vi "Logout_init.vi"(8 "error in (no error)":errorcluster, 11 "ZenGage v3.0 UI in":T1) -> (0 "error out":errorcluster)   [LabVIEW 2019, in "ZenGage v3.0 UI.lvclass"]
uses:
  ZenGage v3.0 UI.lvclass
  <vilib>/Utility/miscctls.llb/LVRowAndColumnTypeDef.ctl
  Type Definitions/Controls and Indicators/Select a part (combobox).ctl
  Type Definitions/Controls and Indicators/EDL control references.ctl
  Type Definitions/Controls and Indicators/Diagnostics control referencs.ctl
  Type Definitions/Controls and Indicators/Inspection control references.ctl
  Type Definitions/Controls and Indicators/General_Control references.ctl
  Type Definitions/Controls and Indicators/Controls and Indicators Cluster.ctl
  Type Definitions/General/Master sample references.ctl
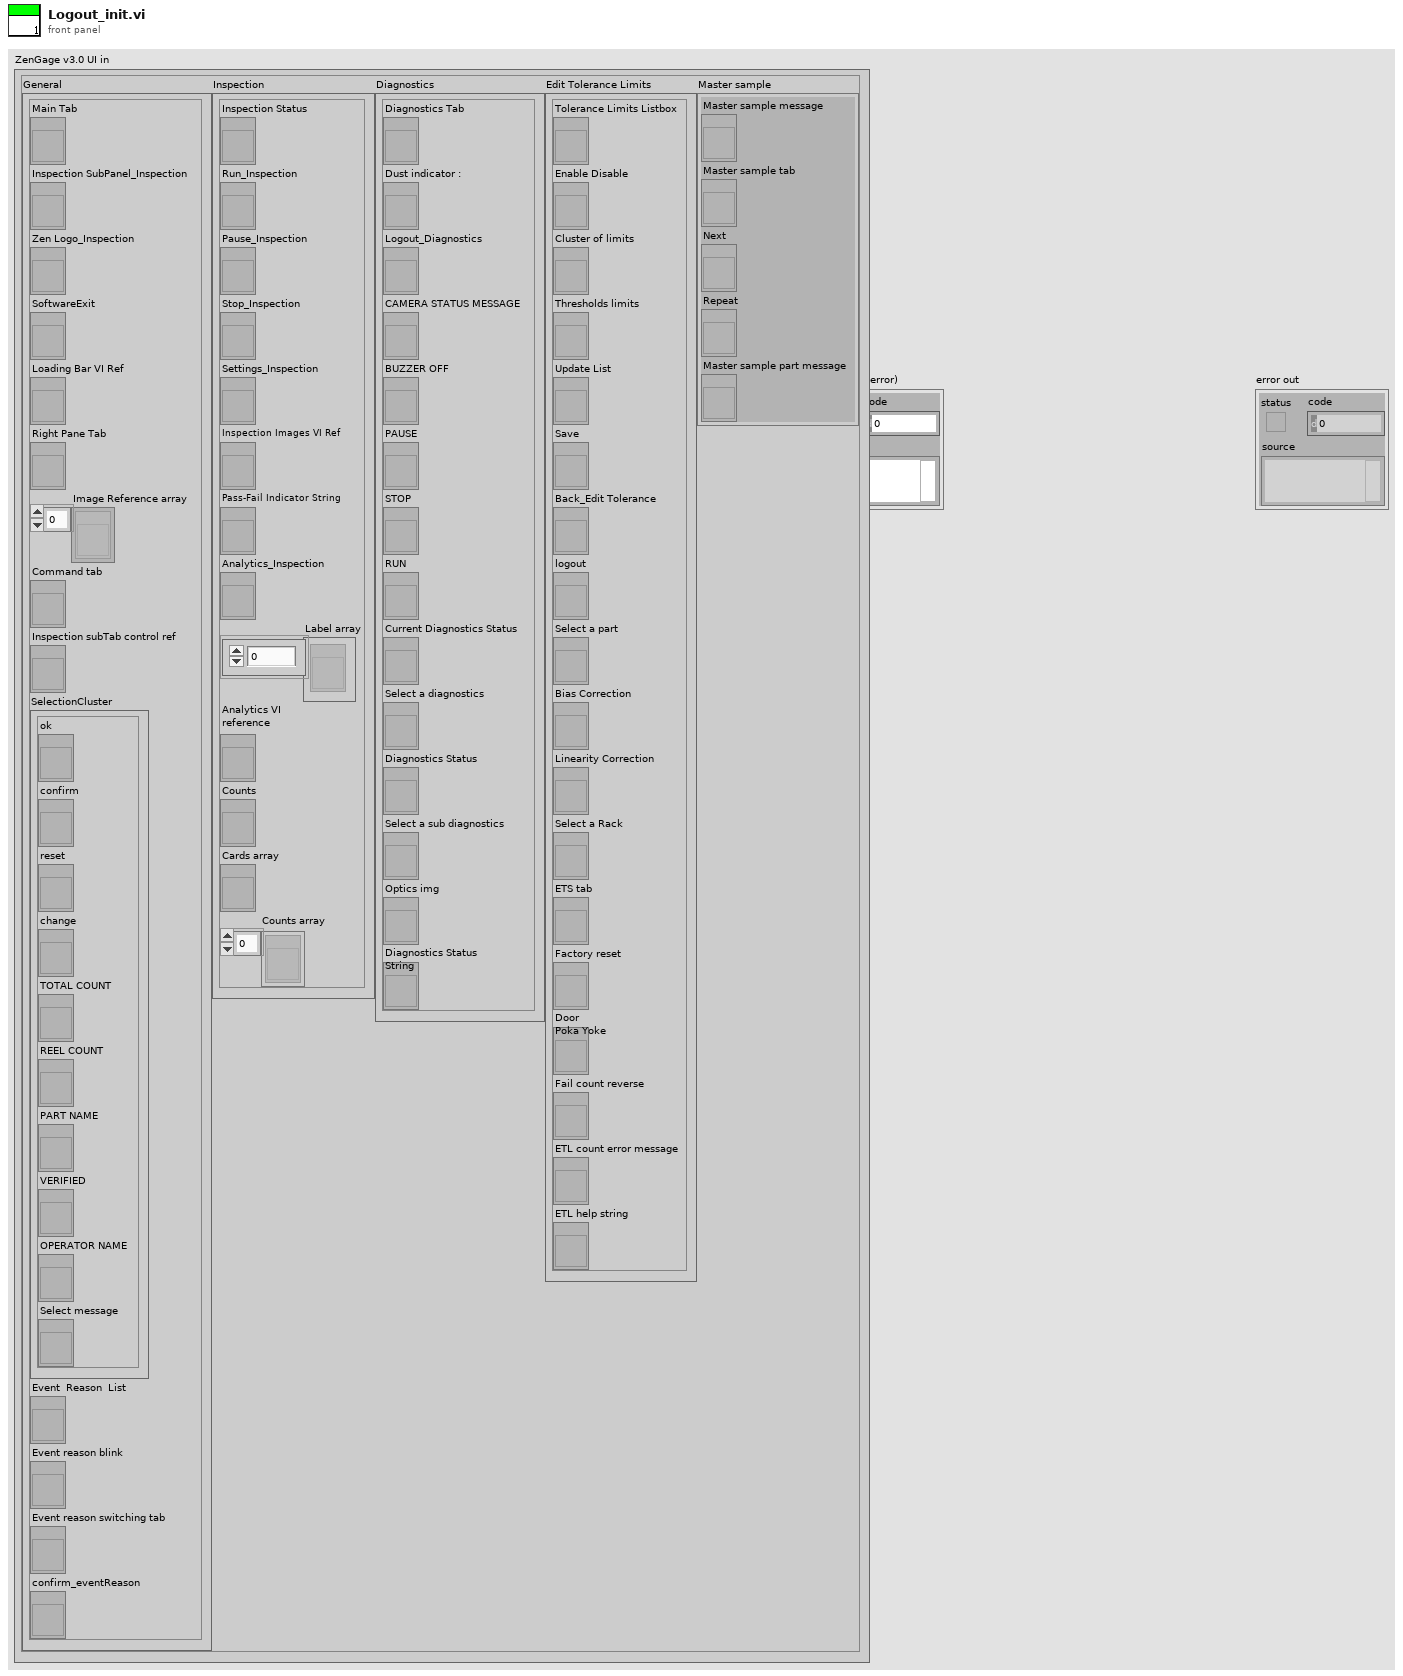
[diagram p1: front panel]
types:
  T1 = typedef "ZenGage v3.0 UI.lvclass/Controls and Indicators Cluster.ctl" = cluster{"General":T2, "Inspection":T3, "Diagnostics":T4, "Edit Tolerance Limits":T5, "Master sample":T6}
  T2 = typedef "ZenGage v3.0 UI.lvclass/General_Control references.ctl" = cluster{"Main Tab":refnum<vi>, "Inspection SubPanel_Inspection":refnum<vi>, "Zen Logo_Inspection":refnum<vi>, "SoftwareExit":refnum<vi>, "Loading Bar VI Ref":refnum<vi>, "Right Pane Tab":refnum<vi>, "Image Reference array":refnum<vi>[], "Command tab":refnum<vi>, "Inspection subTab control ref":refnum<vi>, "SelectionCluster":cluster{"ok":refnum<vi>, "confirm":refnum<vi>, "reset":refnum<vi>, "change":refnum<vi>, "TOTAL COUNT":refnum<vi>, "REEL COUNT":refnum<vi>, "PART NAME":refnum<vi>, "VERIFIED":refnum<vi>, "OPERATOR NAME":refnum<vi>, "Select message":refnum<vi>}, "Event  Reason  List":refnum<vi>, "Event reason blink":refnum<vi>, "Event reason switching tab":refnum<vi>, "confirm_eventReason":refnum<vi>}
  T3 = typedef "ZenGage v3.0 UI.lvclass/Inspection control references.ctl" = cluster{"Inspection Status":refnum<vi>, "Run_Inspection":refnum<vi>, "Pause_Inspection":refnum<vi>, "Stop_Inspection":refnum<vi>, "Settings_Inspection":refnum<vi>, "Inspection Images VI Ref":refnum<vi>, "Pass-Fail Indicator String":refnum<vi>, "Analytics_Inspection":refnum<vi>, "Label array":refnum<vi>[], "Analytics VI\nreference":refnum<vi>, "Counts":refnum<vi>, "Cards array":refnum<vi>, "Counts array":refnum<vi>[]}
  T4 = typedef "ZenGage v3.0 UI.lvclass/Diagnostics control referencs.ctl" = cluster{"Diagnostics Tab":refnum<vi>, "Dust indicator :":refnum<vi>, "Logout_Diagnostics":refnum<vi>, "CAMERA STATUS MESSAGE":refnum<vi>, "BUZZER OFF":refnum<vi>, "PAUSE":refnum<vi>, "STOP":refnum<vi>, "RUN":refnum<vi>, "Current Diagnostics Status":refnum<vi>, "Select a diagnostics":refnum<vi>, "Diagnostics Status":refnum<vi>, "Select a sub diagnostics":refnum<vi>, "Optics img":refnum<vi>, "Diagnostics Status\nString":refnum<vi>}
  T5 = typedef "ZenGage v3.0 UI.lvclass/EDL control references.ctl" = cluster{"Tolerance Limits Listbox":refnum<vi>, "Enable Disable":refnum<vi>, "Cluster of limits":refnum<vi>, "Thresholds limits":refnum<vi>, "Update List":refnum<vi>, "Save":refnum<vi>, "Back_Edit Tolerance":refnum<vi>, "logout":refnum<vi>, "Select a part":refnum<vi>, "Bias Correction":refnum<vi>, "Linearity Correction":refnum<vi>, "Select a Rack":refnum<vi>, "ETS tab":refnum<vi>, "Factory reset":refnum<vi>, "Door\nPoka Yoke":refnum<vi>, "Fail count reverse":refnum<vi>, "ETL count error message":refnum<vi>, "ETL help string":refnum<vi>}
  T6 = typedef "Master sample references.ctl" = cluster{"Master sample message":refnum<vi>, "Master sample tab":refnum<vi>, "Next":refnum<vi>, "Repeat":refnum<vi>, "Master sample part message":refnum<vi>}
  T7 = enum32{"Edit Tolerance Limits1", "Inspection", "Master sample", "Diagnostics"}
  T8 = enum32{"Arduino Motor", "Sensor trigger", "Hardware Button", "Camera Optics"}
  T9 = enum8{"Enabled", "Disabled", "Disabled and Grayed Out"}
  T10 = enum32{"Inspection", "Diagnostics", "Edit Tolerance Settings"}
  T11 = typedef "LVRowAndColumnTypeDef.ctl" = cluster{"Row":i32, "Column":i32}
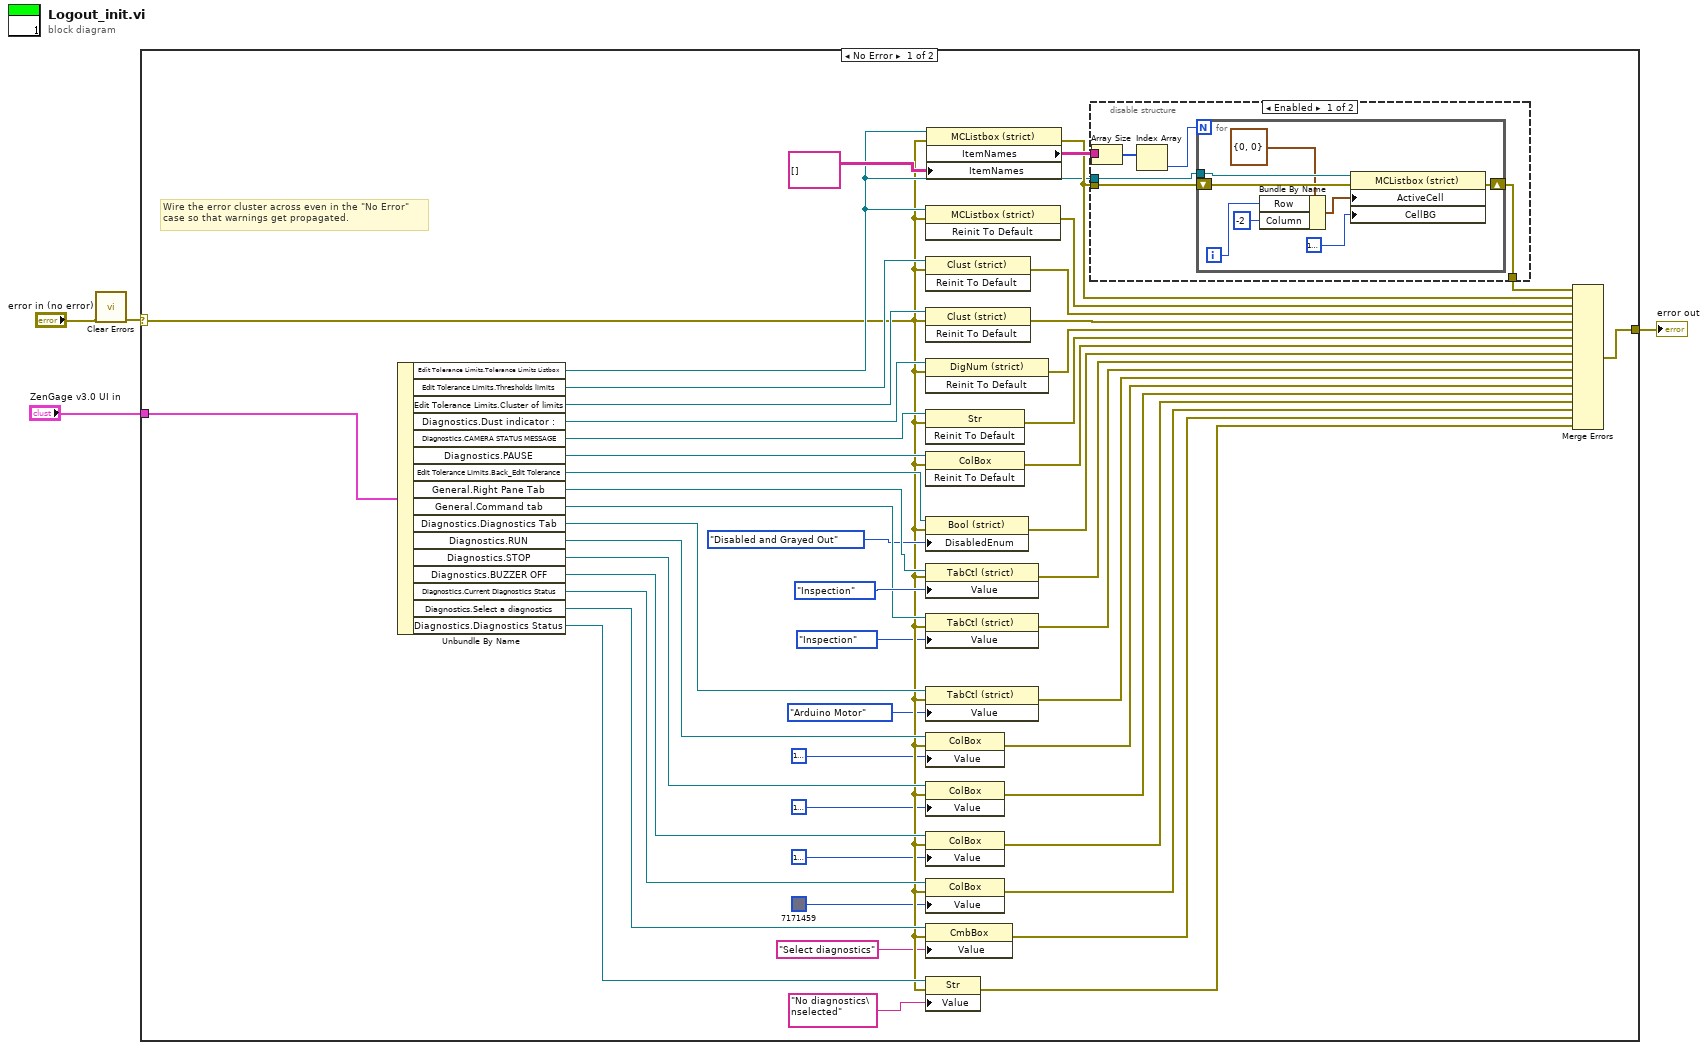
[diagram p0: block diagram]
diagram:
  n1 = call <vilib>:"Clear Errors.vi"("error in (no error)"="error in (no error)") -> ("error out"=w1:errorcluster)  [unwired: 5 in, 1 out]
  n2 = case shown="No Error" w1 {
    selector: w1 -> [w20 w69]
    tunnel: [w40 w69] -> w4
    tunnel: "ZenGage v3.0 UI in" -> [w53 _]
    frame No Error {
      # "Wire the error cluster across even in the \"No Error\"\ncase so that warnings get propagated."
      n3 = Unbundle By Name(w53) -> ("Edit Tolerance Limits.Tolerance Limits Listbox"=w30:refnum<vi>, "Edit Tolerance Limits.Thresholds limits"=w34:refnum<vi>, "Edit Tolerance Limits.Cluster of limits"=w52:refnum<vi>, "Diagnostics.Dust indicator :"=w51:refnum<vi>, "Diagnostics.CAMERA STATUS MESSAGE"=w50:refnum<vi>, "Diagnostics.PAUSE"=w49:refnum<vi>, "Edit Tolerance Limits.Back_Edit Tolerance"=w48:refnum<vi>, "General.Right Pane Tab"=w39:refnum<vi>, "General.Command tab"=w36:refnum<vi>, "Diagnostics.Diagnostics Tab"=w27:refnum<vi>, "Diagnostics.RUN"=w26:refnum<vi>, "Diagnostics.STOP"=w25:refnum<vi>, "Diagnostics.BUZZER OFF"=w24:refnum<vi>, "Diagnostics.Current Diagnostics Status"=w23:refnum<vi>, "Diagnostics.Select a diagnostics"=w22:refnum<vi>, "Diagnostics.Diagnostics Status"=w21:refnum<vi>)
      n4 = invoke class="MCListbox (strict)" method="Reinit To Default"(reference=w30, error in=w20) -> (error out=w47:errorcluster)  [unwired: 1 in, 2 out]
      n5 = invoke class="Clust (strict)" method="Reinit To Default"(reference=w34, error in=w20) -> (error out=w46:errorcluster)  [unwired: 1 in, 2 out]
      n6 = invoke class="Clust (strict)" method="Reinit To Default"(reference=w52, error in=w20) -> (error out=w45:errorcluster)  [unwired: 1 in, 2 out]
      n7 = invoke class="DigNum (strict)" method="Reinit To Default"(reference=w51, error in=w20) -> (error out=w44:errorcluster)  [unwired: 1 in, 2 out]
      n8 = invoke class="Str" method="Reinit To Default"(reference=w50, error in=w20) -> (error out=w43:errorcluster)  [unwired: 1 in, 2 out]
      n9 = invoke class="ColBox" method="Reinit To Default"(reference=w49, error in=w20) -> (error out=w42:errorcluster)  [unwired: 1 in, 2 out]
      n10 = property class="Bool (strict)"(reference=w48, error in=w20, "DisabledEnum"=T9."Disabled and Grayed Out" ("Disabled")) -> (error out=w41:errorcluster)  [unwired: 1 out]
      n11 = property class="TabCtl (strict)"(reference=w39, error in=w20, "Value"=T10."Inspection") -> (error out=w37:errorcluster)  [unwired: 1 out]
      n12 = property class="TabCtl (strict)"(reference=w36, error in=w20, "Value"=T7."Inspection") -> (error out=w35:errorcluster)  [unwired: 1 out]
      n13 = property class="TabCtl (strict)"(reference=w27, error in=w20, "Value"=T8."Arduino Motor") -> (error out=w19:errorcluster)  [unwired: 1 out]
      n14 = property class="ColBox"(reference=w26, error in=w20, "Value"=u32 16777216) -> (error out=w18:errorcluster)  [unwired: 1 out]
      n15 = property class="ColBox"(reference=w25, error in=w20, "Value"=u32 16777216) -> (error out=w17:errorcluster)  [unwired: 1 out]
      n16 = property class="ColBox"(reference=w24, error in=w20, "Value"=u32 16777216) -> (error out=w16:errorcluster)  [unwired: 1 out]
      n17 = property class="ColBox"(reference=w23, error in=w20, "Value"=u32 7171459) -> (error out=w15:errorcluster)  [unwired: 1 out]
      n18 = property class="CmbBox"(reference=w22, error in=w20, "Value"="Select diagnostics") -> (error out=w14:errorcluster)  [unwired: 1 out]
      n19 = property class="Str"(reference=w21, error in=w20, "Value"="No diagnostics\nselected") -> (error out=w13:errorcluster)  [unwired: 1 out]
      n20 = property class="MCListbox (strict)"(reference=w30, error in=w20, "ItemNames"=string[][] [] ("Item Names")) -> (error out=w31:errorcluster, "ItemNames"=w32:string[][])  [unwired: 1 out]
      n21 = disable-structure shown="Enabled" {
        disable-tunnel: w32 -> [w59 _]
        disable-tunnel: w31 -> [w56 w68]
        disable-tunnel: w30 -> [w55 _]
        disable-tunnel: [w54 w68] -> w29
        frame Enabled {
          n22 = Array Size(array=w59) -> (size(s)=w58:i32[])
          n23 = Index Array(array=w58) -> (element=w57:i32)  [unwired: 1 in]
          n24 = for {
            N: w57 -> [_]
            shift-right: [w66] -> w54
            shift-left: w56 -> [w67]
            tunnel: w55 -> [w65]
            i -> [w63]
            n25 = Bundle By Name(cluster=T11 {"Row"=0, "Column"=0} ("Active Cell:Active Cell"), "Row"=w63, "Column"=-2) -> (w61:T11)
            n26 = property class="MCListbox (strict)"(reference=w65, error in=w67, "ActiveCell"=w61, "CellBG"=u32 16777216) -> (error out=w66:errorcluster)  [unwired: 1 out]
          }
        }
        frame Disabled {
        }
      }
      n27 = Merge Errors(w29, w31, w47, w46, w45, w44, w43, w42, w41, w37, w35, w19, w18, w17, w16, w15, w14, w13) -> (w40:errorcluster)
    }
    frame Error {
    }
  }
  "error out" <- w4
